vi "ZSlice compute-core2.vi"(6 "ZStage Pos":dbl, 7 "Objective Pos Locked":bool, 8 "error in (no error)":errorcluster, 9 "ZStep":dbl, 10 "ZStop":dbl, 11 "ZStart":dbl) -> (0 "error out":errorcluster, 1 "Motor Z Planes(um)":dbl[](array[numeric]) format="%#_12f", 2 "# of Z-planes":i32, 3 "AOL Z Planes(um)":dbl[](array[numeric]) format="%#_12f", 5 "ZStagePos":dbl)   [LabVIEW 2020]
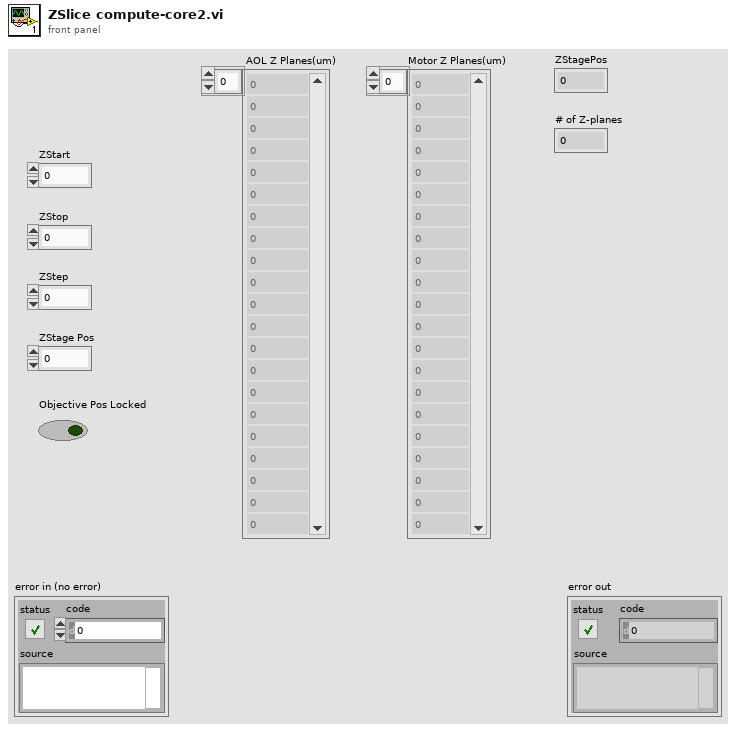
[diagram p1: front panel]
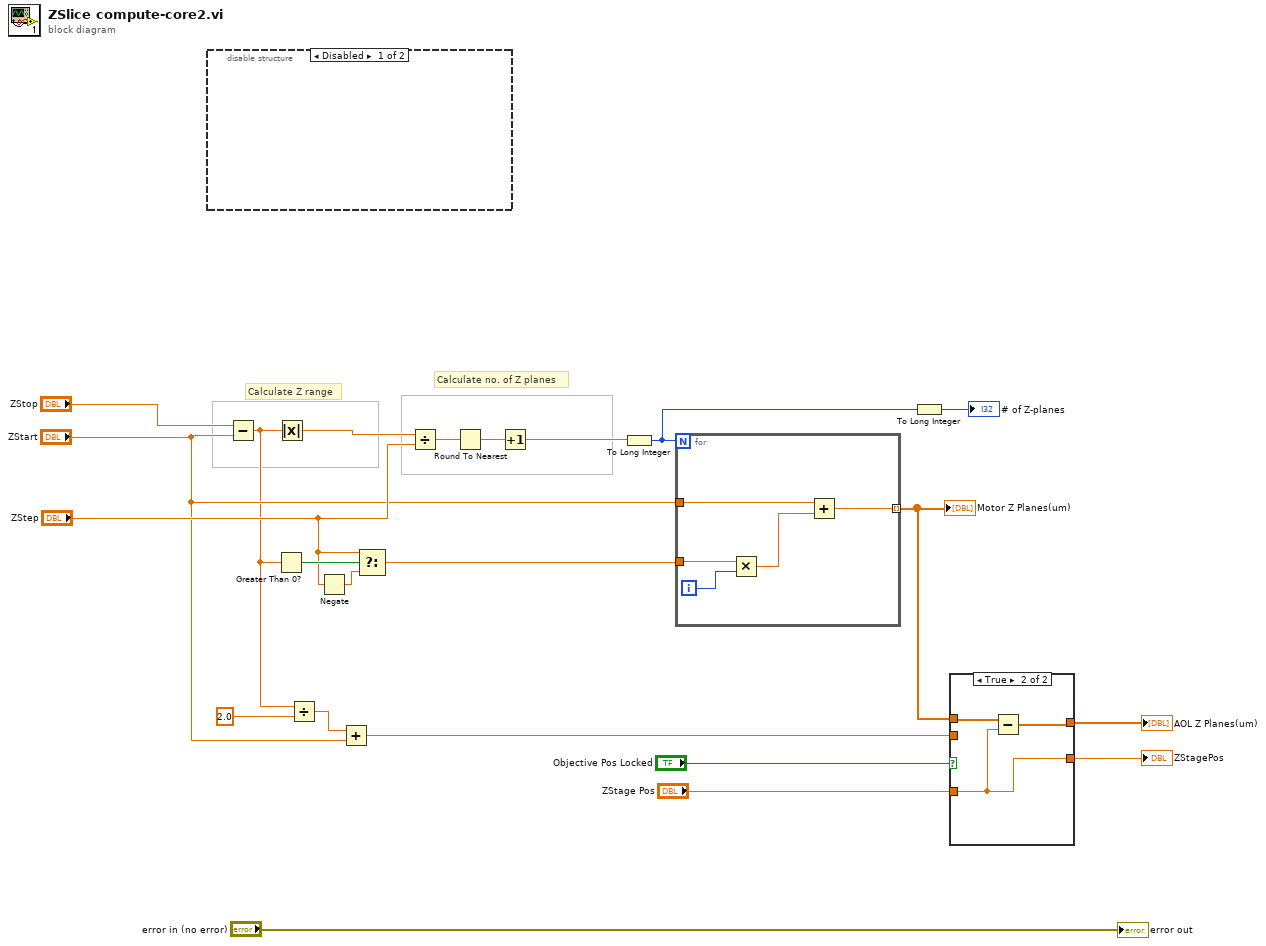
[diagram p0: block diagram]
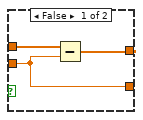
[diagram p2: hidden frame]
diagram:
  # "Calculate no. of Z planes"
  # "Calculate Z range"
  n1 = disable-structure shown="Disabled" {
    frame Disabled {
    }
    frame Enabled {
    }
  }
  n2 = Subtract(x="ZStop", y="ZStart") -> (x-y=w10:dbl)
  n3 = Greater Than 0?(x=w10) -> (x > 0?=w17:bool)
  n4 = Absolute Value(x=w10) -> (abs(x)=w21:dbl)
  n5 = Divide(x=w10, y=2.0) -> (x/y=w8:dbl)
  n6 = Negate(x="ZStep") -> (-x=w15:dbl)
  n7 = Add(x=w8, y="ZStart") -> (x+y=w5:dbl)
  n8 = Select(t="ZStep", s=w17, f=w15) -> (s? t:f=w14:dbl)
  n9 = Divide(x=w21, y="ZStep") -> (x/y=w20:dbl)
  n10 = Round To Nearest(number=w20) -> (nearest integer value=w19:dbl)
  n11 = Increment(x=w19) -> (x+1=w18:dbl)
  n12 = To Long Integer(number=w18) -> (32bit integer=w12:i32)
  n13 = for {
    N: w12 -> [_]
    tunnel: w14 -> [w27]
    tunnel: "ZStart" -> [w25]
    tunnel: [w23] -> w6 mode=indexing
    i -> [w26]
    n14 = Multiply(x=w27, y=w26) -> (x*y=w24:dbl)
    n15 = Add(x=w25, y=w24) -> (x+y=w23:dbl)
  }
  "Motor Z Planes(um)" <- w6
  n16 = To Long Integer(number=w12) -> (32bit integer=→"# of Z-planes":i32)
  n17 = case shown="True" "Objective Pos Locked" {
    tunnel: w6 -> [w30 w33]
    tunnel: w5 -> [w28 _]
    tunnel: [w29 w32] -> w4
    tunnel: [w28 w31] -> w3
    tunnel: "ZStage Pos" -> [_ w31]
    frame False {
      n18 = Subtract(x=w30, y=w28) -> (x-y=w29:dbl[])
    }
    frame True {
      n19 = Subtract(x=w33, y=w31) -> (x-y=w32:dbl[])
    }
  }
  "AOL Z Planes(um)" <- w4
  "ZStagePos" <- w3
  "error out" <- "error in (no error)"
